vi "Stop.vi"(8 "error in (no error)":errorcluster, 10 "Message in":refnum<class "StopMessage.lvclass">, 11 "Tomo in":refnum<class "Tomo.lvclass">) -> (0 "error out":errorcluster, 3 "Tomo out":refnum<class "Tomo.lvclass">)   [LabVIEW 2012, in "Tomo.lvclass"]
doc: "This member function is called when the statemachine in the run.vi receives an 'stop' command. It relays the message to all observers of the component.\n\nOverride this member function in your derived class if you need additional stop functionality (but don't forget to call the parent method)."
uses:
  Tomo.lvclass
  <vilib>/Distrio/Murmex/StopMessage/StopMessage.lvclass
  Current activity.ctl
  Tomo.lvclass/Tomo.ctl
  notice type.ctl
  <vilib>/Distrio/Murmex/Murmex/Murmex.lvclass
panel:
  # "This method is called when the STOP\ntrigger is sent. \n\nOverride this method when your component needs to\nrespond to this trigger. \n\nCall parent for proper implementation"
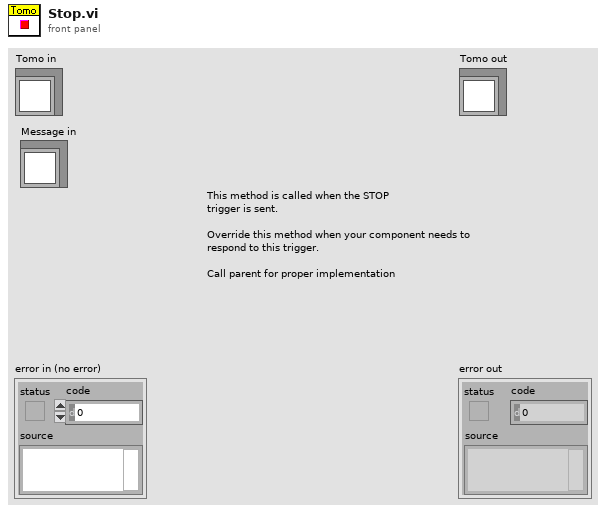
[diagram p1: front panel]
types:
  T1 = typedef "Tomo.lvclass/Current activity.ctl" = enum16{"Idle", "Inter-stack motion", "Pre-tomo calculation", "Stack acquisition", "Stack preparation", "Pre-tomo stack acq", "Pre-tomo inter-stack"}
  T2 = typedef "Tomo.lvclass/notice type.ctl" = enum16{"Tomography stopped", "Tomography error", "Tomography finished", "Timing issue", "Critical timing issue"}
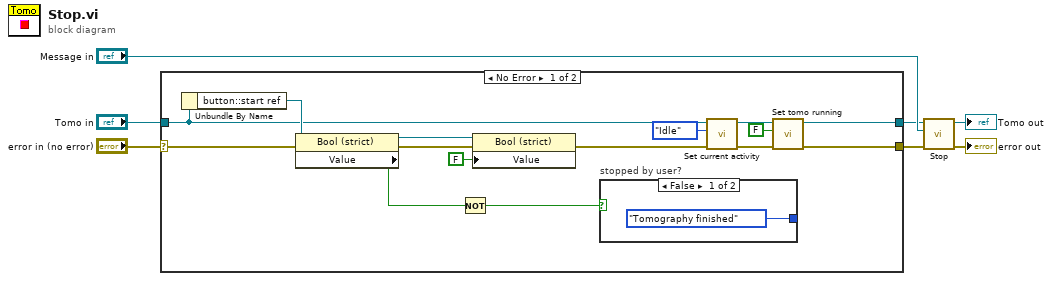
[diagram p0: block diagram]
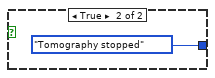
[diagram p2: hidden frame]
diagram:
  n1 = case shown="No Error" "error in (no error)" {
    selector: "error in (no error)" -> [w22 w26]
    tunnel: [w9 w26] -> w3
    tunnel: "Tomo in" -> [w12 w25]
    tunnel: [w8 w25] -> w1
    frame No Error {
      n2 = Unbundle By Name(w12) -> ("button::start ref"=w18:refnum<vi>)
      n3 = property class="Bool (strict)"(reference=w18, error in=w22) -> (reference out=w17:refnum<vi>, error out=w19:errorcluster, "Value"=w16:bool)
      n4 = Not(x=w16) -> (.not. x?=w15:bool)
      n5 = property class="Bool (strict)"(reference=w17, error in=w19, "Value"=FALSE) -> (error out=w13:errorcluster)  [unwired: 1 out]
      n6 = case "stopped by user?" shown="False" w15 {
        tunnel: [notice_type."Tomography finished" ("Notice type") notice_type."Tomography stopped" ("Notice type")] -> _
        frame False {
        }
        frame True {
        }
      }
      n7 = call-dynamic "Set current activity.vi"("error in (no error)"=w13, "Current activity"=Current_activity."Idle", "Tomo in"=w12) -> ("error out"=w14:errorcluster, "Tomo out"=w11:refnum<class "Tomo.lvclass">)  [unwired: 7 in]
      n8 = call-dynamic "Set tomo running.vi"("error in (no error)"=w14, "tomo running?"=FALSE, "Tomo in"=w11) -> ("error out"=w9:errorcluster, "Tomo out"=w8:refnum<class "Tomo.lvclass">)  [unwired: 7 in]
    }
    frame Error {
    }
  }
  n9 = call-parent "Stop.vi"("error in (no error)"=w3, "Message in"="Message in", "Murmex in"=w1) -> ("error out"=→"error out":errorcluster, "Murmex out"=→"Tomo out":refnum<class "Tomo.lvclass">)  [unwired: 7 in]
